vi "Connections.vi"() -> ()   [LabVIEW 2017]
uses:
  <vilib>/Utility/file.llb/Read From Spreadsheet File (I64).vi
  <vilib>/Utility/file.llb/Read From Spreadsheet File (DBL).vi
  <vilib>/Utility/file.llb/Write To Spreadsheet File (string).vi
  <vilib>/Utility/file.llb/Write To Spreadsheet File (DBL).vi
panel:
  out "ArraySens 2":i8[](array[numeric])
  in  "Sensitivity 2":u16(ring) items=["NA", "2 nV", "5 nV", "10 nV", "20 nV", "50 nV", "100 nV", "200 nV", "500 nV", "1 uV", "2 uV", "5 uV", "10 uV", "20 uV", "50 uV", "100 uV", "200 uV", "500 uV", "1 mV", "2 mV", "5 mV", "10 mV", "20 mV", "50 mV", "100 mV", "200 mV", "500 mV", "1 V"]
  in  "Open Existing":bool
  out "ArraySens":i8[](array[numeric])
  out "ArrayOsc":dbl[](array[numeric])
  in  "Oscillator (V)":dbl
  in  "Sensitivity":u16(ring) items=["2 nV", "5 nV", "10 nV", "20 nV", "50 nV", "100 nV", "200 nV", "500 nV", "1 uV", "2 uV", "5 uV", "10 uV", "20 uV", "50 uV", "100 uV", "200 uV", "500 uV", "1 mV", "2 mV", "5 mV", "10 mV", "20 mV", "50 mV", "100 mV", "200 mV", "500 mV", "1 V"]
  in  "Save and Exit":bool
  out "Large Array":bool[][][](array[boolean])
  out "Configuration file:":path
  in  "Config #":u16(ring) items=["Configuration #1", "Configuration #2", "Configuration #3", "Configuration #4"]
  in  "# of Configs":i8=3
  out "Connection file:":path
  out "String":string
  in  "Save":bool
  in  "Table":bool[][](array[boolean])
  out "Array 2":string[](array[string])
  in  "Array":u16[](array[ring]) items=["--", "1", "2", "3", "4", "5", "6", "7", "8", "9", "10", "11", "12", "13", "14", "15", "16", "17", "18", "19", "20", "21", "22", "23", "24", "25", "26", "27"]
  # "(This file stores \"connection\" (2-A; 4-B itc.). Experimental configurations are stored in the file below)"
  # "Oscillator"
  # "NanoVolt Hi"
  # "Lock-In 1 Hi"
  # "Lock-In 2 Hi"
  # "Chan. B Hi"
  # "Total number of \nexperimental \nconfigurations \nto be measured:"
  # "Choose config # and enter connections manually"
  # "\"Configuration\"\nfile:"
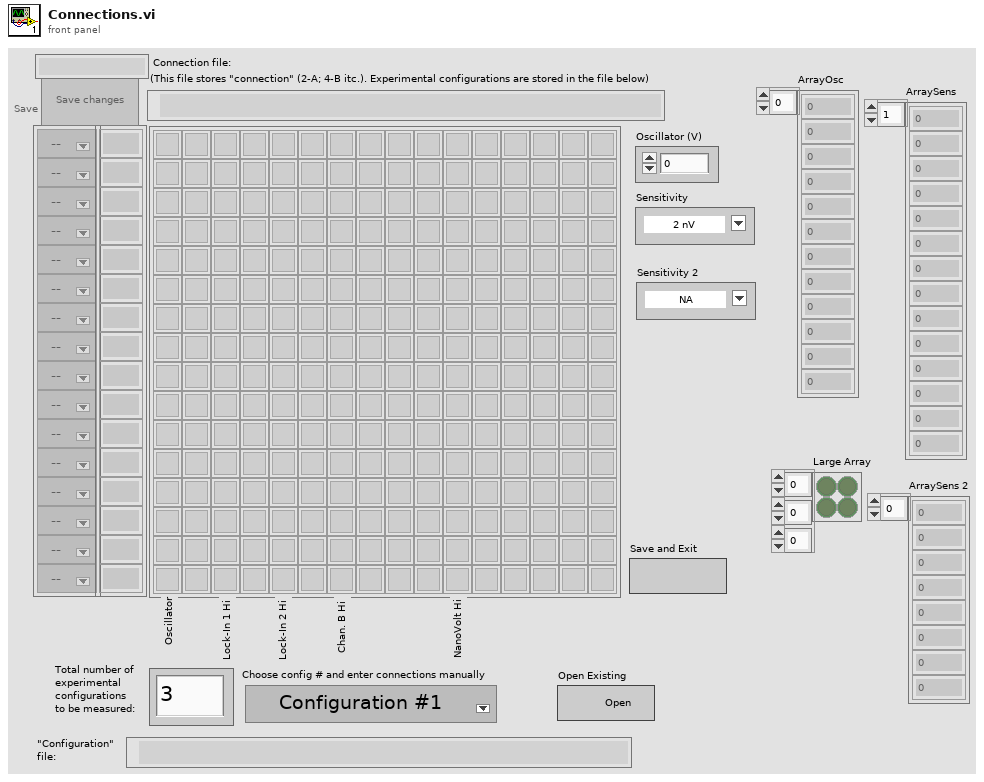
[diagram p1: front panel]
types:
  T1 = enum8{"Enabled", "Disabled", "Disabled and Grayed Out"}
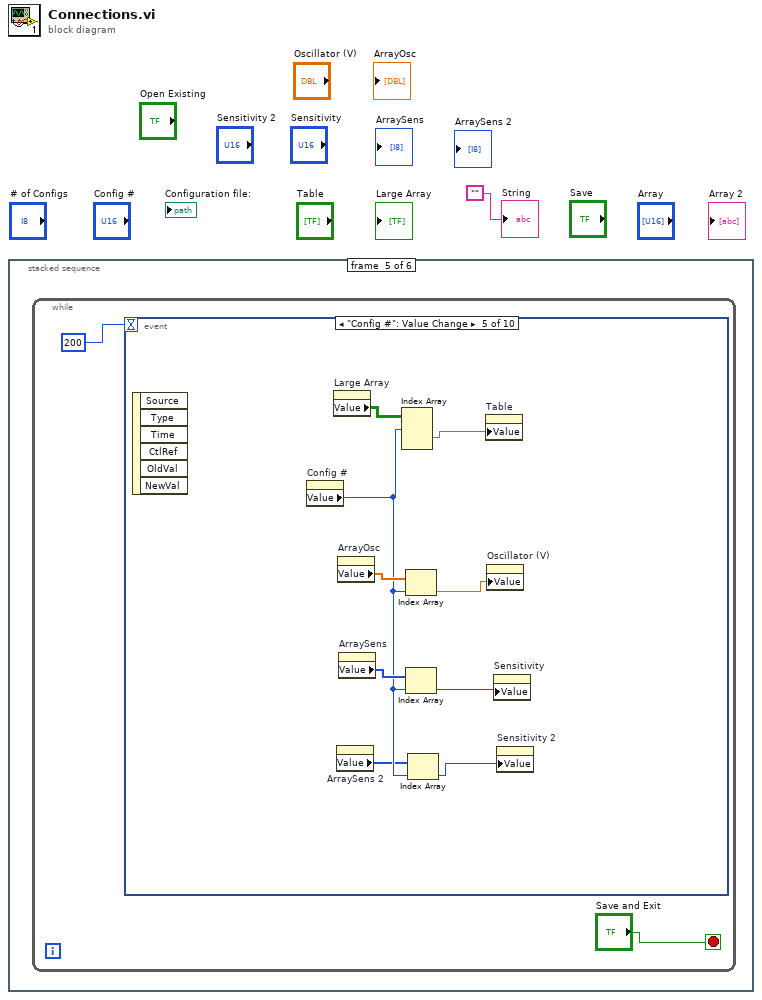
[diagram p0: block diagram]
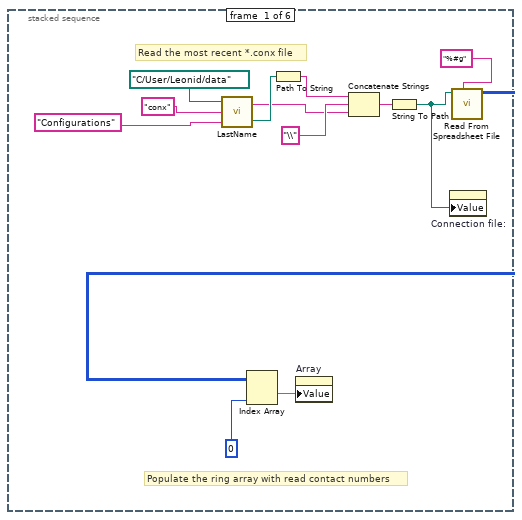
[diagram p2: hidden frame]
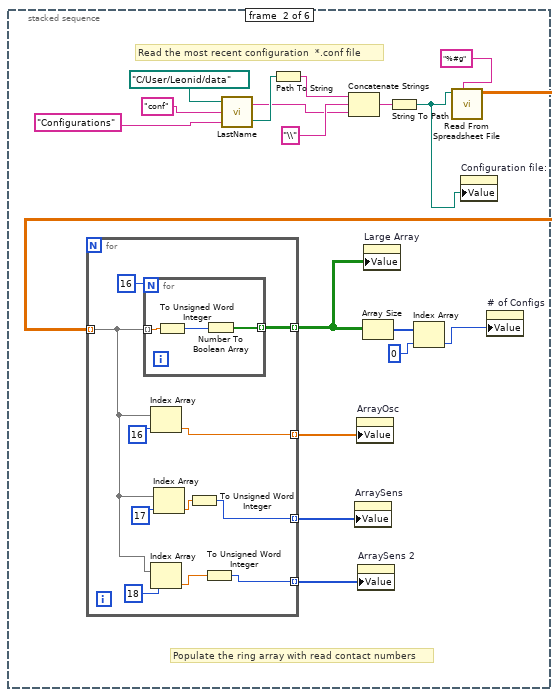
[diagram p3: hidden frame]
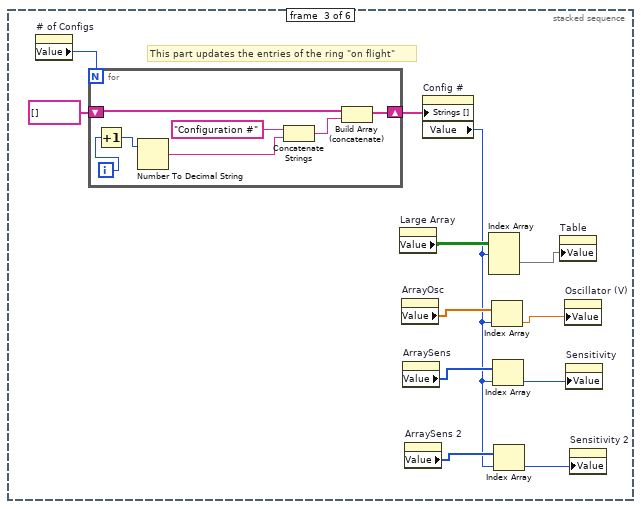
[diagram p4: hidden frame]
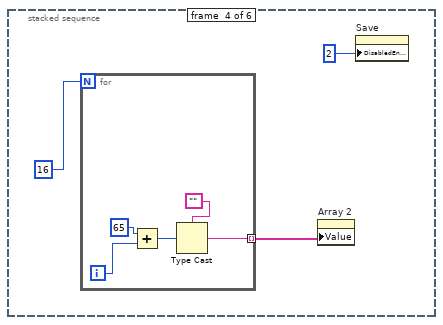
[diagram p5: hidden frame]
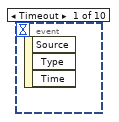
[diagram p6: hidden frame]
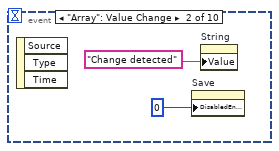
[diagram p7: hidden frame]
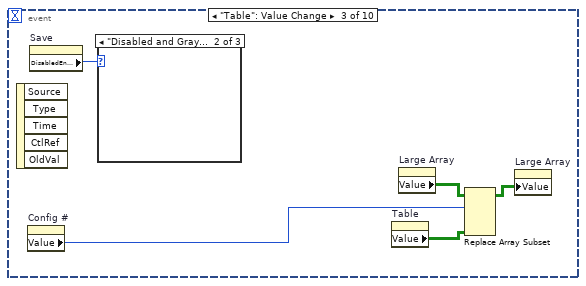
[diagram p8: hidden frame]
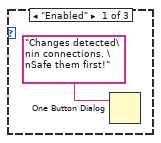
[diagram p9: hidden frame]
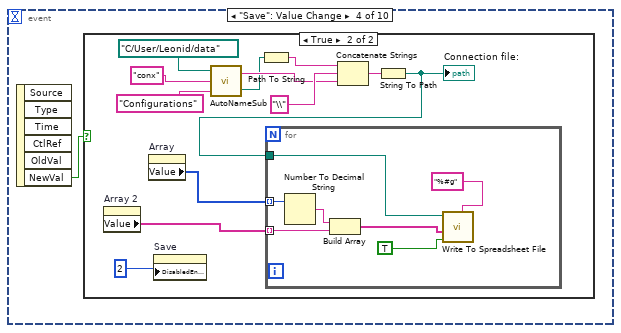
[diagram p11: hidden frame]
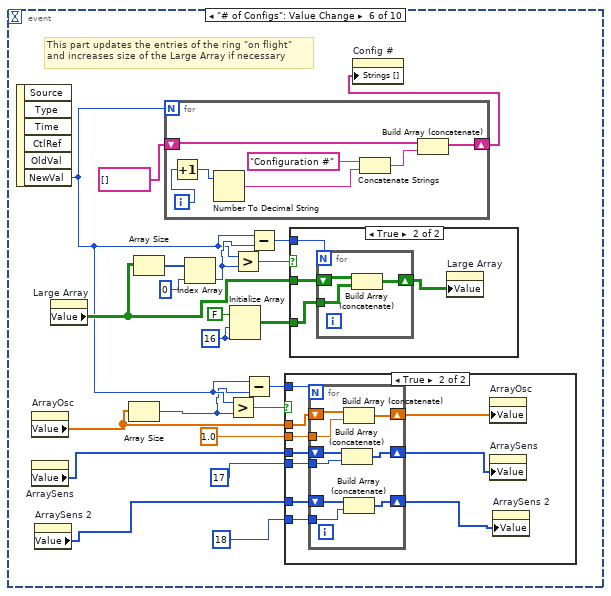
[diagram p13: hidden frame]
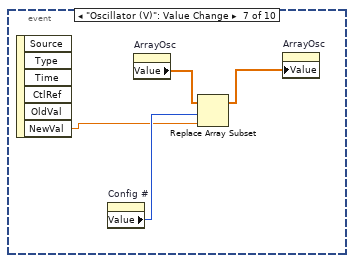
[diagram p16: hidden frame]
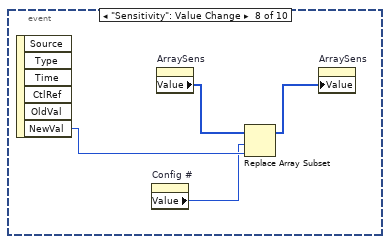
[diagram p17: hidden frame]
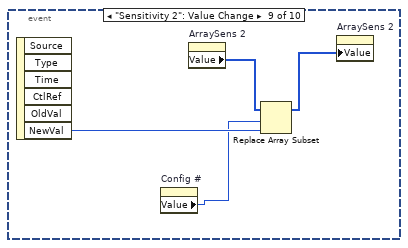
[diagram p18: hidden frame]
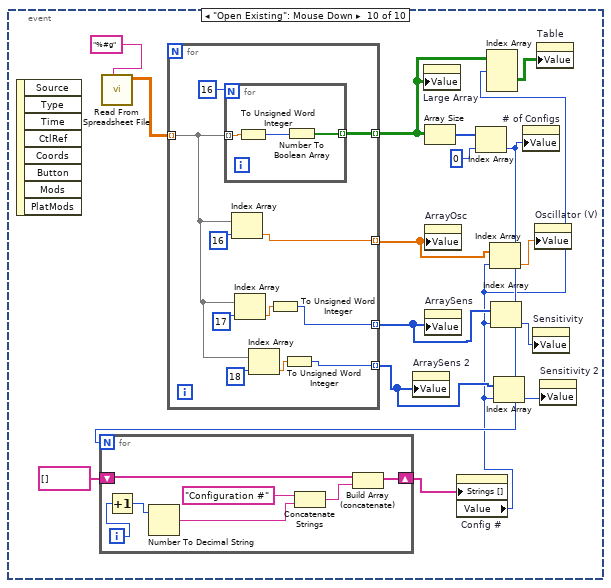
[diagram p19: hidden frame]
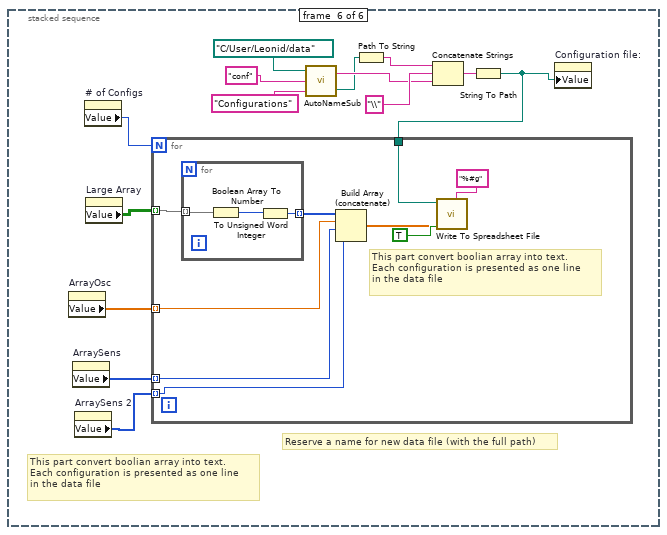
[diagram p20: hidden frame]
diagram:
  n1 = stacked-sequence {
    frame #0 {
      # "Populate the ring array with read contact numbers"
      # "Read the most recent *.conx file"
      n2 = call "LastName.vi"("Custom Folder"="Configurations", "Extention"="conx", "User Data Folder"=path "C:/User/Leonid/data") -> ("created path"=w10:path, "String"=w9:string)
      n3 = Path To String(path=w10) -> (string=w14:string)
      n4 = Concatenate Strings(w14, "\\", w9) -> (w12:string)
      n5 = String To Path(string=w12) -> (path=w2:path)
      n6 = property on="Connection file:" class="Path"("Value"=w2) -> ()  [unwired: 2 in, 2 out]
      n7 = call-poly <vilib>:"Read From Spreadsheet File.vi"("format (%d)"="%#g", "file path (dialog if empty)"=w2) -> ("all rows"=w3:i64[][])  [unwired: 5 in, 4 out]
      n8 = Index Array(array=w3, index (col)=0) -> (element=w5:i64[])  [unwired: 1 in]
      n9 = property on="Array" class="Arr (strict)"("Value"=w5) -> ()  [unwired: 2 in, 2 out]
    }
    frame #1 {
      # "Populate the ring array with read contact numbers"
      # "Read the most recent configuration  *.conf file"
      n10 = call "LastName.vi"("Custom Folder"="Configurations", "Extention"="conf", "User Data Folder"=path "C:/User/Leonid/data") -> ("created path"=w28:path, "String"=w27:string)
      n11 = Path To String(path=w28) -> (string=w32:string)
      n12 = Concatenate Strings(w32, "\\", w27) -> (w30:string)
      n13 = String To Path(string=w30) -> (path=w23:path)
      n14 = call-poly <vilib>:"Read From Spreadsheet File.vi"("format (%.3f)"="%#g", "file path (dialog if empty)"=w23) -> ("all rows"=w22:dbl[][])  [unwired: 5 in, 4 out]
      n15 = for {
        tunnel: w22 -> [w35] mode=indexing
        tunnel: [w43] -> w21 mode=indexing
        tunnel: [w40] -> w17 mode=indexing
        tunnel: [w37] -> w16 mode=indexing
        tunnel: [w33] -> w15 mode=indexing
        n16 = for {
          N: 16 -> [_]
          tunnel: w35 -> [w46] mode=indexing
          tunnel: [w44] -> w43 mode=indexing
          n17 = To Unsigned Word Integer(number=w46) -> (unsigned 16bit integer=w45:u16)
          n18 = Number To Boolean Array(number=w45) -> (Boolean array=w44:bool[])
        }
        n19 = Index Array(array=w35, index=16) -> (element=w40:dbl)
        n20 = Index Array(array=w35, index=18) -> (element=w34:dbl)
        n21 = Index Array(array=w35, index=17) -> (element=w38:dbl)
        n22 = To Unsigned Word Integer(number=w38) -> (unsigned 16bit integer=w37:u16)
        n23 = To Unsigned Word Integer(number=w34) -> (unsigned 16bit integer=w33:u16)
      }
      n24 = property on="ArraySens" class="Arr (strict)"("Value"=w16) -> ()  [unwired: 2 in, 2 out]
      n25 = property on="ArrayOsc" class="Arr (strict)"("Value"=w17) -> ()  [unwired: 2 in, 2 out]
      n26 = property on="ArraySens 2" class="Arr (strict)"("Value"=w15) -> ()  [unwired: 2 in, 2 out]
      n27 = Array Size(array=w21) -> (size(s)=w20:i32[])
      n28 = property on="Large Array" class="Arr (strict)"("Value"=w21) -> ()  [unwired: 2 in, 2 out]
      n29 = Index Array(array=w20, index=0) -> (element=w19:i32)
      n30 = property on="Configuration file:" class="Path"("Value"=w23) -> ()  [unwired: 2 in, 2 out]
      n31 = property on="# of Configs" class="DigNum (strict)"("Value"=w19) -> ()  [unwired: 2 in, 2 out]
    }
    frame #2 {
      # "This part updates the entries of the ring \"on flight\""
      n32 = property on="# of Configs" class="DigNum (strict)"() -> ("Value"=w58:i8)  [unwired: 2 in, 2 out]
      n33 = for {
        N: w58 -> [_]
        shift-right: [w62] -> w57
        shift-left: string[] [] -> [w63]
        i -> [w60]
        n34 = Increment(x=w60) -> (x+1=w59:i32)
        n35 = Number To Decimal String(number=w59) -> (decimal integer string=w64:string)  [unwired: 1 in]
        n36 = Concatenate Strings("Configuration #", w64) -> (w61:string)
        n37 = Build Array (concatenate)(w63, w61) -> (w62:string[])
      }
      n38 = property on="Large Array" class="Arr (strict)"() -> ("Value"=w56:bool[][][])  [unwired: 2 in, 2 out]
      n39 = property on="ArrayOsc" class="Arr (strict)"() -> ("Value"=w53:dbl[])  [unwired: 2 in, 2 out]
      n40 = property on="ArraySens" class="Arr (strict)"() -> ("Value"=w51:i8[])  [unwired: 2 in, 2 out]
      n41 = property on="ArraySens 2" class="Arr (strict)"() -> ("Value"=w49:i8[])  [unwired: 2 in, 2 out]
      n42 = property on="Config #" class="Ring (strict)"("Strings []"=w57) -> ("Value"=w48:u16)  [unwired: 2 in, 2 out]
      n43 = Index Array(array=w56, index (dim 0)=w48) -> (element=w55:bool[][])  [unwired: 2 in]
      n44 = Index Array(array=w53, index=w48) -> (element=w52:dbl)
      n45 = Index Array(array=w51, index=w48) -> (element=w50:i8)
      n46 = Index Array(array=w49, index=w48) -> (element=w47:i8)
      n47 = property on="Table" class="Arr (strict)"("Value"=w55) -> ()  [unwired: 2 in, 2 out]
      n48 = property on="Oscillator (V)" class="DigNum (strict)"("Value"=w52) -> ()  [unwired: 2 in, 2 out]
      n49 = property on="Sensitivity" class="Ring (strict)"("Value"=w50) -> ()  [unwired: 2 in, 2 out]
      n50 = property on="Sensitivity 2" class="Ring (strict)"("Value"=w47) -> ()  [unwired: 2 in, 2 out]
    }
    frame #3 {
      n51 = for {
        N: 16 -> [_]
        tunnel: [w69] -> w67 mode=indexing
        i -> [w72]
        n52 = Add(x=65, y=w72) -> (x+y=w70:i32)
        n53 = Type Cast(type="", x=w70) -> (*(type *) &x=w69:string)
      }
      n54 = property on="Array 2" class="Arr (strict)"("Value"=w67) -> ()  [unwired: 2 in, 2 out]
      n55 = property on="Save" class="Bool"("DisabledEnum"=2) -> ()  [unwired: 2 in, 2 out]
    }
    frame #4 {
      n56 = while {
        stop <- "Save and Exit" stop-if-true
        n57 = event shown="[4] \"Config #\": Value Change" {
          selector: _ -> [_ _ _ _ _ _ _ _ _ _]
          dyn-events: _ -> [_ _ _ _ _ _ _ _ _ _]
          timeout: 200 -> [_ _ _ _ _ _ _ _ _ _]
          event Timeout {
            n58 = event-data() -> ()  [unwired: 1 in, 3 out]
          }
          event "Array": Value Change {
            n59 = event-data() -> ()  [unwired: 1 in, 3 out]
            n60 = property on="Save" class="Bool"("DisabledEnum"=0) -> ()  [unwired: 2 in, 2 out]
            n61 = property on="String" class="Str"("Value"="Change detected") -> ()  [unwired: 2 in, 2 out]
          }
          event "Table": Value Change {
            n62 = event-data() -> ()  [unwired: 1 in, 5 out]
            n63 = property on="Config #" class="Ring (strict)"() -> ("Value"=w79:u16)  [unwired: 2 in, 2 out]
            n64 = property on="Save" class="Bool"() -> ("DisabledEnum"=w82:T1)  [unwired: 2 in, 2 out]
            n65 = case shown="\"Disabled and Grayed Out\", Default" w82 {
              frame "Enabled" {
                n66 = One Button Dialog(message="Changes detected\nin connections. \nSafe them first!") -> ()  [unwired: 1 in, 1 out]
              }
              frame "Disabled and Grayed Out", Default {
              }
              frame "Disabled" {
              }
            }
            n67 = property on="Table" class="Arr (strict)"() -> ("Value"=w78:bool[][])  [unwired: 2 in, 2 out]
            n68 = property on="Large Array" class="Arr (strict)"() -> ("Value"=w81:bool[][][])  [unwired: 2 in, 2 out]
            n69 = Replace Array Subset(array=w81, new element=w78, index (dim 0)=w79) -> (w80:bool[][][])  [unwired: 2 in]
            n70 = property on="Large Array" class="Arr (strict)"("Value"=w80) -> ()  [unwired: 2 in, 2 out]
          }
          event "Save": Value Change {
            n71 = event-data() -> ("NewVal"=w84:bool)  [unwired: 1 in, 5 out]
            n72 = case shown="True" w84 {
              frame False {
              }
              frame True {
                n73 = property on="Array 2" class="Arr (strict)"() -> ("Value"=w95:string[])  [unwired: 2 in, 2 out]
                n74 = property on="Array" class="Arr (strict)"() -> ("Value"=w96:u16[])  [unwired: 2 in, 2 out]
                n75 = property on="Save" class="Bool"("DisabledEnum"=2) -> ()  [unwired: 2 in, 2 out]
                n76 = call "AutoNameSub.vi"("Custom Folder"="Configurations", "Extention"="conx", "User Data Folder"=path "C:/User/Leonid/data") -> ("created path"=w86:path, "String"=w91:string)  [unwired: 1 in]
                n77 = Path To String(path=w86) -> (string=w87:string)
                n78 = Concatenate Strings(w87, "\\", w91) -> (w93:string)
                n79 = String To Path(string=w93) -> (path=w88:path)
                "Connection file:" <- w88
                n80 = for {
                  tunnel: w96 -> [w101] mode=indexing
                  tunnel: w95 -> [w99] mode=indexing
                  tunnel: w88 -> [w97]
                  n81 = Number To Decimal String(number=w101) -> (decimal integer string=w100:string)  [unwired: 1 in]
                  n82 = Build Array(w100, w99) -> (w98:string[])
                  n83 = call-poly <vilib>:"Write To Spreadsheet File.vi"("format (%s)"="%#g", "append to file? (new file:F)"=TRUE, "1D data"=w98, "file path (dialog if empty)"=w97) -> ()  [unwired: 4 in, 1 out]
                }
              }
            }
          }
          event "Config #": Value Change {
            n84 = event-data() -> ()  [unwired: 1 in, 6 out]
            n85 = property on="Config #" class="Ring (strict)"() -> ("Value"=w106:u16)  [unwired: 2 in, 2 out]
            n86 = property on="Large Array" class="Arr (strict)"() -> ("Value"=w112:bool[][][])  [unwired: 2 in, 2 out]
            n87 = property on="ArraySens 2" class="Arr (strict)"() -> ("Value"=w105:i8[])  [unwired: 2 in, 2 out]
            n88 = property on="ArrayOsc" class="Arr (strict)"() -> ("Value"=w110:dbl[])  [unwired: 2 in, 2 out]
            n89 = property on="ArraySens" class="Arr (strict)"() -> ("Value"=w108:i8[])  [unwired: 2 in, 2 out]
            n90 = Index Array(array=w112, index (dim 0)=w106) -> (element=w111:bool[][])  [unwired: 2 in]
            n91 = Index Array(array=w110, index=w106) -> (element=w109:dbl)
            n92 = Index Array(array=w108, index=w106) -> (element=w107:i8)
            n93 = Index Array(array=w105, index=w106) -> (element=w104:i8)
            n94 = property on="Table" class="Arr (strict)"("Value"=w111) -> ()  [unwired: 2 in, 2 out]
            n95 = property on="Oscillator (V)" class="DigNum (strict)"("Value"=w109) -> ()  [unwired: 2 in, 2 out]
            n96 = property on="Sensitivity" class="Ring (strict)"("Value"=w107) -> ()  [unwired: 2 in, 2 out]
            n97 = property on="Sensitivity 2" class="Ring (strict)"("Value"=w104) -> ()  [unwired: 2 in, 2 out]
          }
          event "# of Configs": Value Change {
            w126 = 16
            # "This part updates the entries of the ring \"on flight\"\nand increases size of the Large Array if necessary"
            n98 = event-data() -> ("NewVal"=w119:i8)  [unwired: 1 in, 5 out]
            n99 = property on="ArrayOsc" class="Arr (strict)"() -> ("Value"=w120:dbl[])  [unwired: 2 in, 2 out]
            n100 = property on="ArraySens" class="Arr (strict)"() -> ("Value"=w116:i8[])  [unwired: 2 in, 2 out]
            n101 = property on="ArraySens 2" class="Arr (strict)"() -> ("Value"=w114:i8[])  [unwired: 2 in, 2 out]
            n102 = property on="Large Array" class="Arr (strict)"() -> ("Value"=w123:bool[][][])  [unwired: 2 in, 2 out]
            n103 = Array Size(array=w120) -> (size(s)=w118:i32)
            n104 = Array Size(array=w123) -> (size(s)=w131:i32[])
            n105 = for {
              N: w119 -> [_]
              shift-right: [w163] -> w132
              shift-left: string[] [] -> [w164]
              i -> [w161]
              n106 = Increment(x=w161) -> (x+1=w160:i32)
              n107 = Number To Decimal String(number=w160) -> (decimal integer string=w165:string)  [unwired: 1 in]
              n108 = Concatenate Strings("Configuration #", w165) -> (w162:string)
              n109 = Build Array (concatenate)(w164, w162) -> (w163:string[])
            }
            n110 = Index Array(array=w131, index=0) -> (element=w128:i32)
            n111 = Greater?(x=w119, y=w118) -> (0:w122:bool)
            n112 = Initialize Array(FALSE, w126, w126) -> (w124:bool[][])
            n113 = Greater?(x=w119, y=w128) -> (0:w129:bool)
            n114 = Subtract(x=w119, y=w118) -> (x-y=w121:i32)
            n115 = Subtract(x=w119, y=w128) -> (x-y=w127:i32)
            n116 = case shown="True" w122 {
              tunnel: w121 -> [_ w143]
              tunnel: 1.0 -> [_ w142]
              tunnel: w120 -> [_ w141]
              tunnel: w116 -> [_ w139]
              tunnel: 17 -> [_ w137]
              tunnel: w114 -> [_ w136]
              tunnel: 18 -> [_ w135]
              frame False {
              }
              frame True {
                n117 = for {
                  N: w143 -> [_]
                  shift-right: [w151] -> w140
                  shift-left: w141 -> [w152]
                  shift-right: [w148] -> w138
                  shift-left: w139 -> [w149]
                  tunnel: w142 -> [w150]
                  tunnel: w137 -> [w147]
                  shift-right: [w145] -> w134
                  shift-left: w136 -> [w146]
                  tunnel: w135 -> [w144]
                  n118 = Build Array (concatenate)(w149, w147) -> (w148:i32[])
                  n119 = Build Array (concatenate)(w152, w150) -> (w151:dbl[])
                  n120 = Build Array (concatenate)(w146, w144) -> (w145:i32[])
                }
                n121 = property on="ArrayOsc" class="Arr (strict)"("Value"=w140) -> ()  [unwired: 2 in, 2 out]
                n122 = property on="ArraySens" class="Arr (strict)"("Value"=w138) -> ()  [unwired: 2 in, 2 out]
                n123 = property on="ArraySens 2" class="Arr (strict)"("Value"=w134) -> ()  [unwired: 2 in, 2 out]
              }
            }
            n124 = case shown="True" w129 {
              tunnel: w127 -> [_ w156]
              tunnel: w124 -> [_ w155]
              tunnel: w123 -> [_ w154]
              frame False {
              }
              frame True {
                n125 = for {
                  N: w156 -> [_]
                  shift-right: [w158] -> w153
                  shift-left: w154 -> [w159]
                  tunnel: w155 -> [w157]
                  n126 = Build Array (concatenate)(w159, w157) -> (w158:bool[][][])
                }
                n127 = property on="Large Array" class="Arr (strict)"("Value"=w153) -> ()  [unwired: 2 in, 2 out]
              }
            }
            n128 = property on="Config #" class="Ring (strict)"("Strings []"=w132) -> ()  [unwired: 2 in, 2 out]
          }
          event "Oscillator (V)": Value Change {
            n129 = event-data() -> ("NewVal"=w167:dbl)  [unwired: 1 in, 5 out]
            n130 = property on="Config #" class="Ring (strict)"() -> ("Value"=w168:u16)  [unwired: 2 in, 2 out]
            n131 = property on="ArrayOsc" class="Arr (strict)"() -> ("Value"=w170:dbl[])  [unwired: 2 in, 2 out]
            n132 = Replace Array Subset(array=w170, new element=w167, index=w168) -> (w169:dbl[])
            n133 = property on="ArrayOsc" class="Arr (strict)"("Value"=w169) -> ()  [unwired: 2 in, 2 out]
          }
          event "Sensitivity": Value Change {
            n134 = event-data() -> ("NewVal"=w172:u16)  [unwired: 1 in, 5 out]
            n135 = property on="Config #" class="Ring (strict)"() -> ("Value"=w171:u16)  [unwired: 2 in, 2 out]
            n136 = property on="ArraySens" class="Arr (strict)"() -> ("Value"=w174:i8[])  [unwired: 2 in, 2 out]
            n137 = Replace Array Subset(array=w174, new element=w172, index=w171) -> (w173:i8[])
            n138 = property on="ArraySens" class="Arr (strict)"("Value"=w173) -> ()  [unwired: 2 in, 2 out]
          }
          event "Sensitivity 2": Value Change {
            n139 = event-data() -> ("NewVal"=w178:u16)  [unwired: 1 in, 5 out]
            n140 = property on="Config #" class="Ring (strict)"() -> ("Value"=w177:u16)  [unwired: 2 in, 2 out]
            n141 = property on="ArraySens 2" class="Arr (strict)"() -> ("Value"=w176:i8[])  [unwired: 2 in, 2 out]
            n142 = Replace Array Subset(array=w176, new element=w178, index=w177) -> (w175:i8[])
            n143 = property on="ArraySens 2" class="Arr (strict)"("Value"=w175) -> ()  [unwired: 2 in, 2 out]
          }
          event "Open Existing": Mouse Down {
            n144 = event-data() -> ()  [unwired: 1 in, 8 out]
            n145 = call-poly <vilib>:"Read From Spreadsheet File.vi"("format (%.3f)"="%#g") -> ("all rows"=w193:dbl[][])  [unwired: 6 in, 4 out]
            n146 = for {
              tunnel: w193 -> [w203] mode=indexing
              tunnel: [w212] -> w187 mode=indexing
              tunnel: [w209] -> w185 mode=indexing
              tunnel: [w206] -> w184 mode=indexing
              tunnel: [w202] -> w181 mode=indexing
              n147 = for {
                N: 16 -> [_]
                tunnel: w203 -> [w215] mode=indexing
                tunnel: [w213] -> w212 mode=indexing
                n148 = To Unsigned Word Integer(number=w215) -> (unsigned 16bit integer=w214:u16)
                n149 = Number To Boolean Array(number=w214) -> (Boolean array=w213:bool[])
              }
              n150 = Index Array(array=w203, index=16) -> (element=w209:dbl)
              n151 = Index Array(array=w203, index=17) -> (element=w207:dbl)
              n152 = Index Array(array=w203, index=18) -> (element=w204:dbl)
              n153 = To Unsigned Word Integer(number=w207) -> (unsigned 16bit integer=w206:u16)
              n154 = To Unsigned Word Integer(number=w204) -> (unsigned 16bit integer=w202:u16)
            }
            n155 = property on="ArraySens 2" class="Arr (strict)"("Value"=w181) -> ()  [unwired: 2 in, 2 out]
            n156 = property on="Large Array" class="Arr (strict)"("Value"=w187) -> ()  [unwired: 2 in, 2 out]
            n157 = Array Size(array=w187) -> (size(s)=w192:i32[])
            n158 = property on="ArrayOsc" class="Arr (strict)"("Value"=w185) -> ()  [unwired: 2 in, 2 out]
            n159 = property on="ArraySens" class="Arr (strict)"("Value"=w184) -> ()  [unwired: 2 in, 2 out]
            n160 = Index Array(array=w192, index=0) -> (element=w189:i32)
            n161 = for {
              N: w189 -> [_]
              shift-right: [w198] -> w188
              shift-left: string[] [] -> [w199]
              i -> [w196]
              n162 = Increment(x=w196) -> (x+1=w195:i32)
              n163 = Number To Decimal String(number=w195) -> (decimal integer string=w200:string)  [unwired: 1 in]
              n164 = Concatenate Strings("Configuration #", w200) -> (w197:string)
              n165 = Build Array (concatenate)(w199, w197) -> (w198:string[])
            }
            n166 = property on="Config #" class="Ring (strict)"("Strings []"=w188) -> ("Value"=w180:u16)  [unwired: 2 in, 2 out]
            n167 = Index Array(array=w187, index (dim 0)=w180) -> (element=w186:bool[][])  [unwired: 2 in]
            n168 = Index Array(array=w185, index=w180) -> (element=w183:dbl)
            n169 = Index Array(array=w184, index=w180) -> (element=w182:u16)
            n170 = Index Array(array=w181, index=w180) -> (element=w179:u16)
            n171 = property on="# of Configs" class="DigNum (strict)"("Value"=w189) -> ()  [unwired: 2 in, 2 out]
            n172 = property on="Sensitivity" class="Ring (strict)"("Value"=w182) -> ()  [unwired: 2 in, 2 out]
            n173 = property on="Oscillator (V)" class="DigNum (strict)"("Value"=w183) -> ()  [unwired: 2 in, 2 out]
            n174 = property on="Table" class="Arr (strict)"("Value"=w186) -> ()  [unwired: 2 in, 2 out]
            n175 = property on="Sensitivity 2" class="Ring (strict)"("Value"=w179) -> ()  [unwired: 2 in, 2 out]
          }
        }
      }
    }
    frame #5 {
      # "Reserve a name for new data file (with the full path)"
      # "This part convert boolian array into text. \nEach configuration is presented as one line \nin the data file"
      n176 = property on="ArrayOsc" class="Arr (strict)"() -> ("Value"=w218:dbl[])  [unwired: 2 in, 2 out]
      n177 = property on="ArraySens" class="Arr (strict)"() -> ("Value"=w217:i8[])  [unwired: 2 in, 2 out]
      n178 = property on="ArraySens 2" class="Arr (strict)"() -> ("Value"=w216:i8[])  [unwired: 2 in, 2 out]
      n179 = property on="# of Configs" class="DigNum (strict)"() -> ("Value"=w229:i8)  [unwired: 2 in, 2 out]
      n180 = property on="Large Array" class="Arr (strict)"() -> ("Value"=w228:bool[][][])  [unwired: 2 in, 2 out]
      n181 = call "AutoNameSub.vi"("Custom Folder"="Configurations", "Extention"="conf", "User Data Folder"=path "C:/User/Leonid/data") -> ("created path"=w220:path, "String"=w224:string)  [unwired: 1 in]
      n182 = Path To String(path=w220) -> (string=w221:string)
      n183 = Concatenate Strings(w221, "\\", w224) -> (w226:string)
      n184 = String To Path(string=w226) -> (path=w219:path)
      n185 = for {
        N: w229 -> [_]
        tunnel: w228 -> [w236] mode=indexing
        tunnel: w219 -> [w235]
        tunnel: w218 -> [w232] mode=indexing
        tunnel: w217 -> [w231] mode=indexing
        tunnel: w216 -> [w230] mode=indexing
        # "This part convert boolian array into text. \nEach configuration is presented as one line \nin the data file"
        n186 = for {
          tunnel: [w240] -> w234 mode=indexing
          tunnel: w236 -> [w239] mode=indexing
          n187 = Boolean Array To Number(Boolean array=w239) -> (number=w241:u32)
          n188 = To Unsigned Word Integer(number=w241) -> (unsigned 16bit integer=w240:u16)
        }
        n189 = Build Array (concatenate)(w234, w232, w231, w230) -> (w233:dbl[])
        n190 = call-poly <vilib>:"Write To Spreadsheet File.vi"("format (%.3f)"="%#g", "append to file? (new file:F)"=TRUE, "1D data"=w233, "file path (dialog if empty)"=w235) -> ()  [unwired: 4 in, 1 out]
      }
      n191 = property on="Configuration file:" class="Path"("Value"=w219) -> ()  [unwired: 2 in, 2 out]
    }
  }
  "String" <- ""
